vi "get escaping rate.vi"(7 "TA or MQT":bool, 8 "error in (no error)":errorcluster, 10 "current":dbl, 11 "path in":path) -> (0 "error out":errorcluster, 2 "rate":dbl, 3 "path out":path)   [LabVIEW 2023]
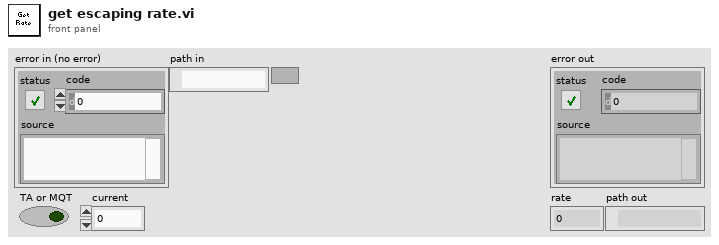
[diagram p1: front panel]
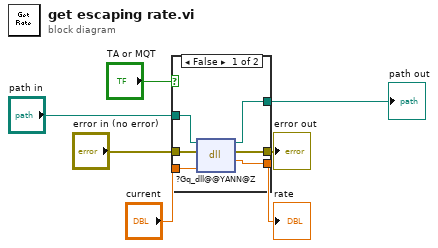
[diagram p0: block diagram]
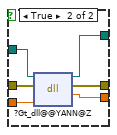
[diagram p2: hidden frame]
diagram:
  n1 = case shown="False" "TA or MQT" {
    tunnel: "error in (no error)" -> [w13 w19]
    tunnel: [w12 w18] -> w6
    tunnel: "current" -> [w11 w17]
    tunnel: [w10 w16] -> w3
    tunnel: "path in" -> [w9 w15]
    tunnel: [w8 w14] -> w1
    frame False {
      n2 = dll-call lib="C:/Users/gyue/Box/Guang Yue uiuc research box folder/computation/Labview simulation GUI/ygDLL.dll" fn="?Gq_dll@@YANN@Z"(path in=w9, error in=w13, "current"=w11) -> (path out=w8:path, error out=w12:errorcluster, "return type"=w10:dbl)  [unwired: 2 in]
    }
    frame True {
      n3 = dll-call lib="C:/Users/gyue/Box/Guang Yue uiuc research box folder/computation/Labview simulation GUI/ygDLL.dll" fn="?Gt_dll@@YANN@Z"(path in=w15, error in=w19, "current"=w17) -> (path out=w14:path, error out=w18:errorcluster, "return type"=w16:dbl)  [unwired: 2 in]
    }
  }
  "error out" <- w6
  "rate" <- w3
  "path out" <- w1
